vi "FRA_UDP_get_timestamp_msg_type.vi"(11 "incoming_UDP":u8[](array[numeric])) -> (0 "end?":bool, 1 "MSG_type_byte":u8, 2 "Time Stamp":timestamp, 3 "datagram_rest":u8[](array[numeric]), 5 "Datagram number":u32)   [LabVIEW 2013]
doc: "Parses UDP dattagram and outputs message type. Dest of the datagram is put to datagram rest."
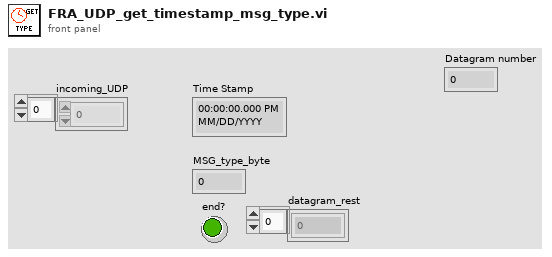
[diagram p1: front panel]
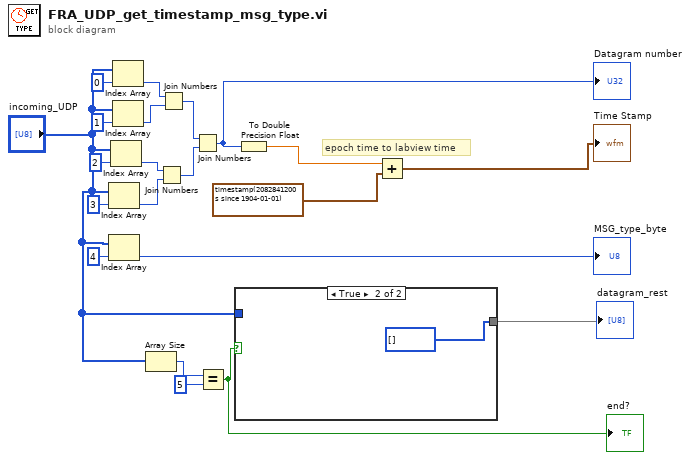
[diagram p0: block diagram]
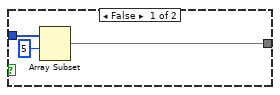
[diagram p2: hidden frame]
diagram:
  # "epoch time to labview time"
  n1 = Index Array(array="incoming_UDP", index=3) -> (element=w15:u8)
  n2 = Index Array(array="incoming_UDP", index=4) -> (element=→"MSG_type_byte":u8)
  n3 = Index Array(array="incoming_UDP", index=2) -> (element=w16:u8)
  n4 = Index Array(array="incoming_UDP", index=0) -> (element=w18:u8)
  n5 = Index Array(array="incoming_UDP", index=1) -> (element=w17:u8)
  n6 = Array Size(array="incoming_UDP") -> (size(s)=w8:i32)
  n7 = Join Numbers(hi=w16, lo=w15) -> ((hi.lo)=w19:u16)
  n8 = Join Numbers(hi=w18, lo=w17) -> ((hi.lo)=w20:u16)
  n9 = Join Numbers(hi=w20, lo=w19) -> ((hi.lo)=w4:u32)
  "Datagram number" <- w4
  n10 = Equal?(x=w8, y=5) -> (x = y?=w6:bool)
  "end?" <- w6
  n11 = case shown="True" w6 {
    tunnel: [w23 u8[] [] ("incoming_UDP")] -> w10
    tunnel: "incoming_UDP" -> [w22 _]
    frame False {
      n12 = Array Subset(array=w22, index=5) -> (w23:u8[])  [unwired: 1 in]
    }
    frame True {
    }
  }
  "datagram_rest" <- w10
  n13 = To Double Precision Float(number=w4) -> (double precision float=w2:dbl)
  n14 = Add(x=w2, y=timestamp(2082841200 s since 1904-01-01) ("current time")) -> (x+y=→"Time Stamp":timestamp)
